vi "Post-Build Custom Action.vi"(10 "Variant":variant) -> (0 "error out":errorcluster)   [LabVIEW 2020]
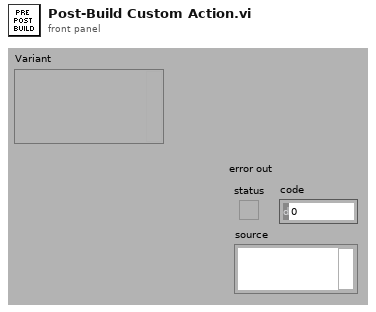
[diagram p1: front panel]
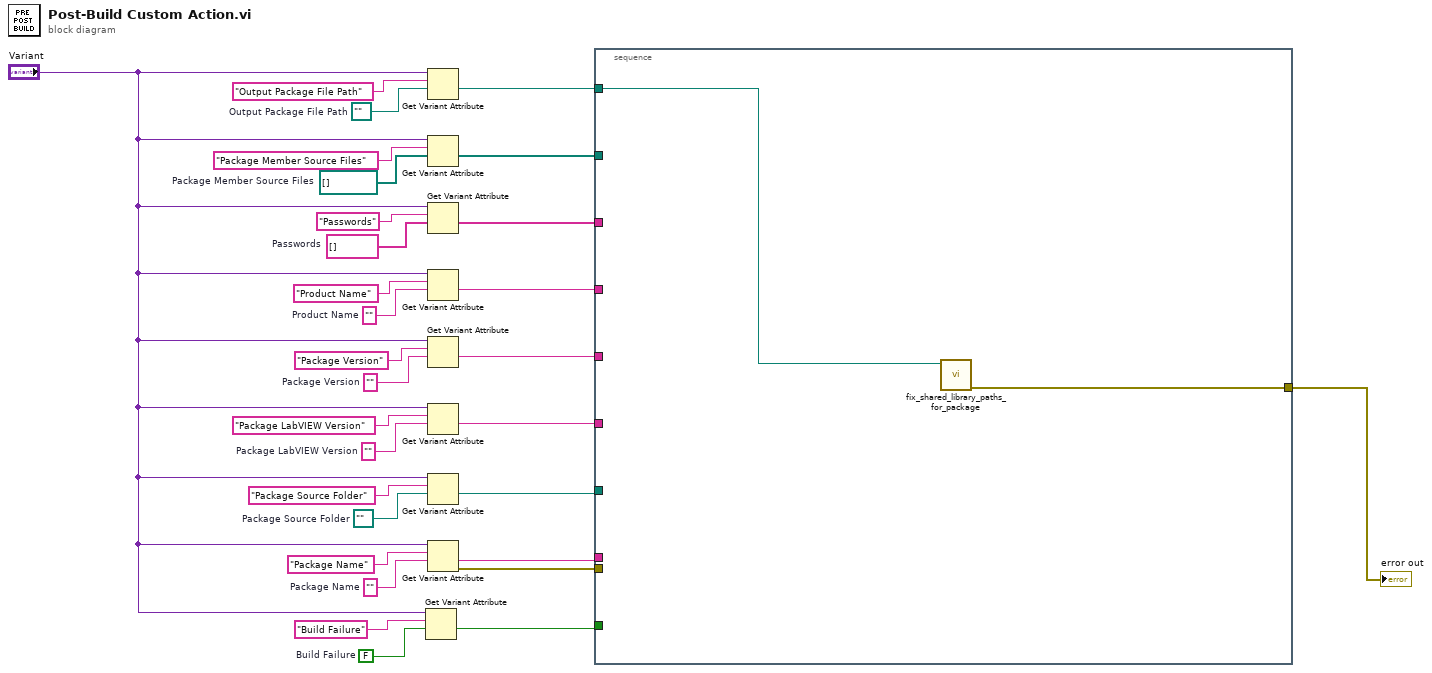
[diagram p0: block diagram]
diagram:
  w5 = FALSE  # Build Failure
  w15 = path ""  # Package Source Folder
  w16 = ""  # Package Name
  w19 = ""  # Package LabVIEW Version
  w21 = ""  # Package Version
  w23 = ""  # Product Name
  w25 = string[] []  # Passwords
  w27 = path[] []  # Package Member Source Files
  w29 = path ""  # Output Package File Path
  n1 = Get Variant Attribute(Variant="Variant", name="Build Failure", default value (empty Variant)=w5) -> (value=w3:bool)  [unwired: 1 in, 3 out]
  n2 = Get Variant Attribute(Variant="Variant", name="Output Package File Path", default value (empty Variant)=w29) -> (value=w14:path)  [unwired: 1 in, 3 out]
  n3 = Get Variant Attribute(Variant="Variant", name="Package Member Source Files", default value (empty Variant)=w27) -> (value=w13:path[])  [unwired: 1 in, 3 out]
  n4 = Get Variant Attribute(Variant="Variant", name="Passwords", default value (empty Variant)=w25) -> (value=w12:string[])  [unwired: 1 in, 3 out]
  n5 = Get Variant Attribute(Variant="Variant", name="Product Name", default value (empty Variant)=w23) -> (value=w11:string)  [unwired: 1 in, 3 out]
  n6 = Get Variant Attribute(Variant="Variant", name="Package Version", default value (empty Variant)=w21) -> (value=w10:string)  [unwired: 1 in, 3 out]
  n7 = Get Variant Attribute(Variant="Variant", name="Package LabVIEW Version", default value (empty Variant)=w19) -> (value=w9:string)  [unwired: 1 in, 3 out]
  n8 = Get Variant Attribute(Variant="Variant", name="Package Source Folder", default value (empty Variant)=w15) -> (value=w8:path)  [unwired: 1 in, 3 out]
  n9 = Get Variant Attribute(Variant="Variant", name="Package Name", default value (empty Variant)=w16) -> (value=w7:string, error out=w1:errorcluster)  [unwired: 1 in, 2 out]
  n10 = stacked-sequence {
    tunnel: w14 -> [w32]
    tunnel: w13 -> [_]
    tunnel: w12 -> [_]
    tunnel: w11 -> [_]
    tunnel: w10 -> [_]
    tunnel: w9 -> [_]
    tunnel: w8 -> [_]
    tunnel: w7 -> [_]
    tunnel: w3 -> [_]
    tunnel: [w31] -> w2
    tunnel: w1 -> [_]
    frame #0 {
      n11 = call "fix_shared_library_paths_for_package.vi"("Package File Path"=w32) -> ("error out"=w31:errorcluster)  [unwired: 10 in]
    }
  }
  "error out" <- w2
